vi "Check mtcdt check gps.vi"(6 "VISA resource name":refnum<visa-resource-name>="COM5", 7 "Passed so far":bool, 8 "error in (no error)":errorcluster) -> (0 "error out":errorcluster, 3 "Response 3":string, 4 "VISA Refnum out":refnum<visa-resource-name>, 5 "Passed?":bool)   [LabVIEW 2024]
panel:
  out "Keyword found index":i32
  out "Response":string
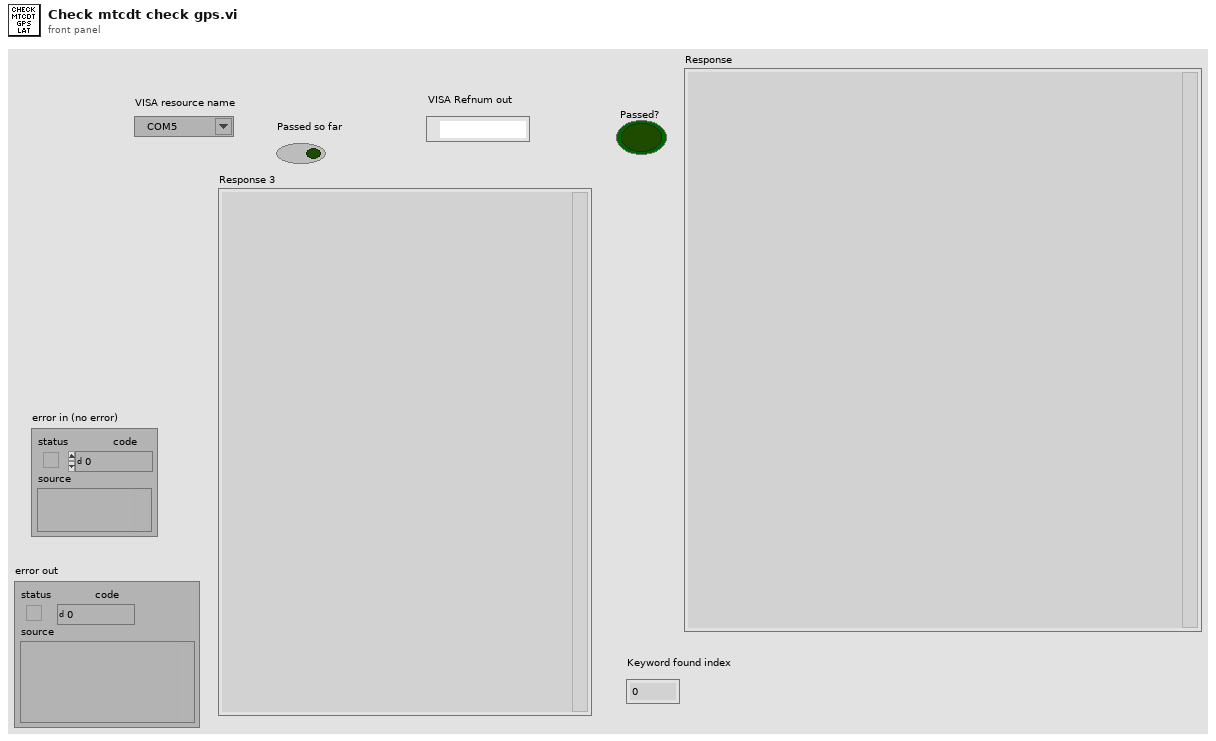
[diagram p1: front panel]
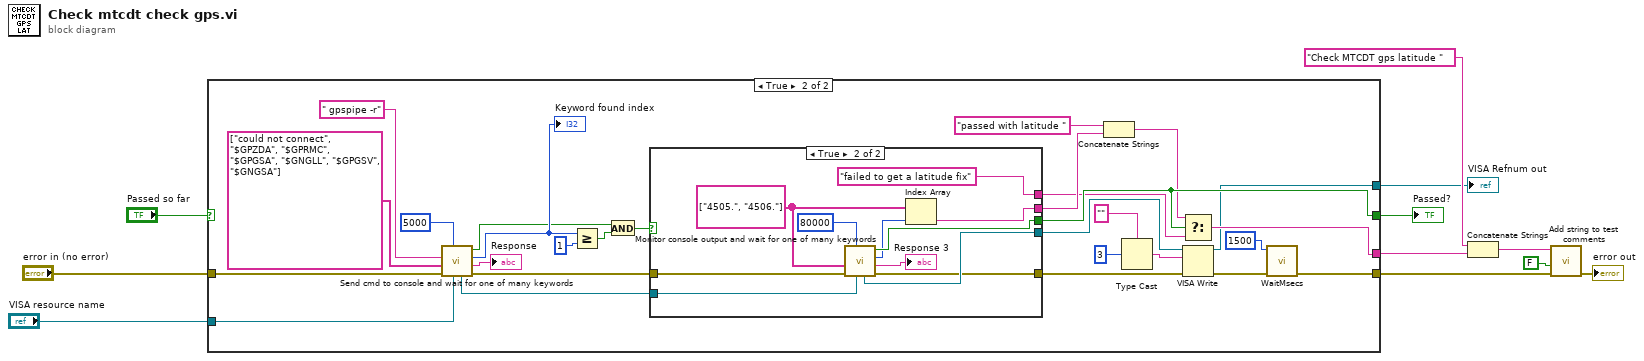
[diagram p0: block diagram]
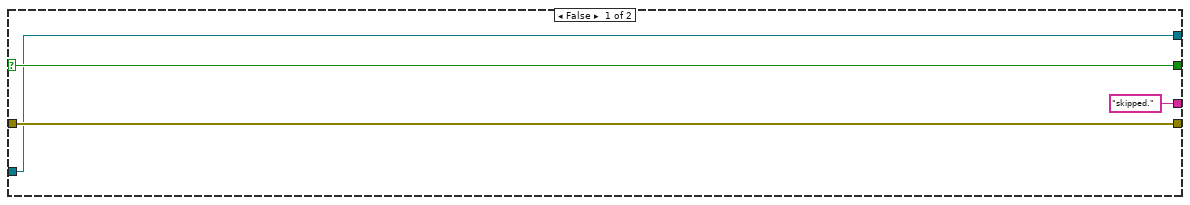
[diagram p2: hidden frame]
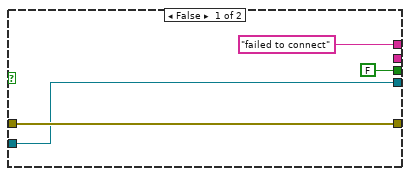
[diagram p3: hidden frame]
diagram:
  n1 = case shown="True" "Passed so far" {
    selector: "Passed so far" -> [w15 _]
    tunnel: "error in (no error)" -> [w14 w40]
    tunnel: [w14 w24] -> w1
    tunnel: "VISA resource name" -> [w13 w38]
    tunnel: [w15 w25] -> w6
    tunnel: [w13 w23] -> w4
    tunnel: ["skipped." w39] -> w5
    frame False {
    }
    frame True {
      n2 = call "Send cmd to console and wait for one of many keywords.vi"("VISA resource name"=w38, "Timeout (1000 mSecs)"=u32 5000, "error in (no error)"=w40, "Wait for keywords"=string[] ["could not connect", "$GPZDA", "$GPRMC", "$GPGSA", "$GNGLL", "$GPGSV", "$GNGSA"], "cmd"=" gpspipe -r") -> ("error out"=w34:errorcluster, "Response"=→"Response":string, "Keyword found index"=w36:i32, "Found key?"=w22:bool, "VISA Refnum out"=w33:refnum<visa-resource-name>)  [unwired: 2 in]
      "Keyword found index" <- w36
      n3 = Greater Or Equal?(x=w36, y=1) -> (x >= y?=w21:bool)
      n4 = And(x=w22, y=w21) -> (x .and. y?=w20:bool)
      n5 = case shown="True" w20 {
        tunnel: w34 -> [w46 w58]
        tunnel: w33 -> [w45 w57]
        tunnel: [w45 w55] -> w29
        tunnel: [w46 w54] -> w28
        tunnel: [FALSE ("Found key?") w52] -> w25
        tunnel: [_ w49] -> w18
        tunnel: ["failed to connect" "failed to get a latitude fix"] -> w16
        frame False {
        }
        frame True {
          w51 = string[] ["4505.", "4506."] ("Wait for keywords")
          n6 = call "Monitor console output and wait for one of many keywords.vi"("VISA resource name"=w57, "Timeout (1000 mSecs)"=u32 80000, "error in (no error)"=w58, "Wait for keywords"=w51) -> ("error out"=w54:errorcluster, "Response"=→"Response 3":string, "Keyword found index"=w50:i32, "Found key?"=w52:bool, "VISA Refnum out"=w55:refnum<visa-resource-name>)  [unwired: 3 in]
          n7 = Index Array(array=w51, index=w50) -> (element=w49:string)
        }
      }
      n8 = Concatenate Strings("passed with latitude ", w18) -> (w17:string)
      n9 = Type Cast(type="", x=3) -> (*(type *) &x=w30:string)
      n10 = Select(t=w17, s=w25, f=w16) -> (s? t:f=w39:string)
      n11 = VISA Write(VISA resource name=w29, write buffer=w30, error in (no error)=w28) -> (VISA resource name out=w23:refnum<visa-resource-name>, error out=w27:errorcluster)  [unwired: 1 out]
      n12 = call "WaitMsecs.vi"("error in (no error)"=w27, "Wait Msecs"=u32 1500) -> ("error out"=w24:errorcluster)  [unwired: 9 in]
    }
  }
  "Passed?" <- w6
  "VISA Refnum out" <- w4
  n13 = Concatenate Strings("Check MTCDT gps latitude " ("string"), w5) -> (w9:string)
  n14 = call "Add string to test comments.vi"("error in (no error)"=w1, "New Section (y)?"=FALSE, "Comments"=w9) -> ("error out"=→"error out":errorcluster)  [unwired: 7 in, 1 out]
